vi "Init CAN Drive.vi"(0 "Front Left Motor Device Number":u8=1, 1 "refnum name":string="robotDrive", 2 "Encoder Codes Per Rev":u16=250, 5 "Rear Left Motor Device Number":u8=2, 7 "Front Right Motor Device Number":u8=3, 9 "Rear Right Motor Device Number":u8=4, 11 "error in (no error)":errorcluster, 12 "Invert":bool=TRUE) -> (15 "error out":errorcluster)   [LabVIEW 2012]
uses:
  <vilib>/Rock Robotics/WPI/CAN/Jaguar/SubVIs/WPI_CANJaguar_ControlMode.ctl
  <vilib>/Rock Robotics/WPI/CAN/Jaguar/SubVIs/WPI_CANJaguar_BrakeCoastMode.ctl
  <vilib>/Rock Robotics/WPI/CAN/Jaguar/SubVIs/WPI_CANJaguar_SpeedReference.ctl
  <vilib>/Rock Robotics/WPI/SafetyOutput/WPI_SafetyOutputConfigMenu.ctl
  <vilib>/Rock Robotics/WPI/MotorControl/WPI_MotorControlOpenCANJaguar.vi
  <vilib>/Rock Robotics/WPI/RobotDrive/WPI_RobotDriveOpen4MotorWithExistingMotors.vi
panel:
  in  "Control Mode":T1
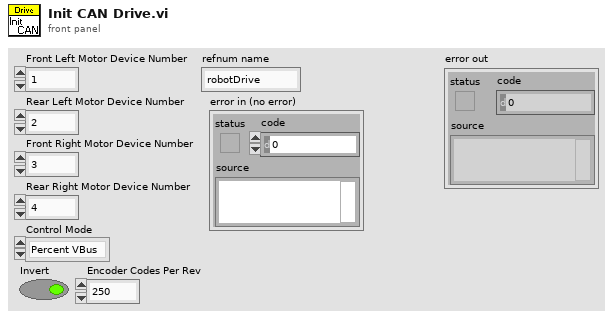
[diagram p1: front panel]
types:
  T1 = typedef "WPI_CANJaguar_ControlMode.ctl" = enum8{"Percent VBus", "Current", "Speed", "Position", "Voltage"}
  T2 = typedef "WPI_SafetyOutputConfigMenu.ctl" = enum16{"Enable", "Disable"}
  T3 = typedef "WPI_CANJaguar_SpeedReference.ctl" = u8
  T4 = typedef "WPI_CANJaguar_BrakeCoastMode.ctl" = enum8{"Jumper", "Brake", "Coast"}
  T5 = typedef "WPI_MotorControlDeviceRef.ctl" = cluster{"DeviceStatus":errorcluster, "Type":enum16{"PWM", "CAN"}, "PWM":cluster{"Digital Module":T6, "PWM Channel":T7, "DeadBand":T8}, "CAN":cluster{"Device Number":u8, "Control Mode":T1, "Semaphore":T9, "Max Vout":dbl}, "Invert":bool, "TransformRef":T10, "InvTransformRef":T10}
  T6 = typedef "FPGA_TypedefDigitalModule.ctl" = enum16{"Digital Module 1", "Digital Module 2"}
  T7 = typedef "FPGA_DIOPWMChannel.ctl" = enum8{"PWM 1", "PWM 2", "PWM 3", "PWM 4", "PWM 5", "PWM 6", "PWM 7", "PWM 8", "PWM 9", "PWM 10", "Invalid"}
  T8 = typedef "WPI_PWMDeadband.ctl" = cluster{"Name":string, "maxPositivePwm":i32, "minPositivePwm":i32, "centerPwm":i32, "maxNegativePwm":i32, "minNegativePwm":i32, "angularRange":u16}
  T9 = typedef "Semaphore RefNum" = refnum<k1>
  T10 = typedef "WPI_PWMTransform_ConPane.ctl" = refnum<vi>
  T11 = typedef "WPI_RobotDriveDevRef.ctl" = cluster{"DevStatus":errorcluster, "Motors[]":T5[], "Square Inputs":bool, "Max Output":dbl, "Isochronous":bool}
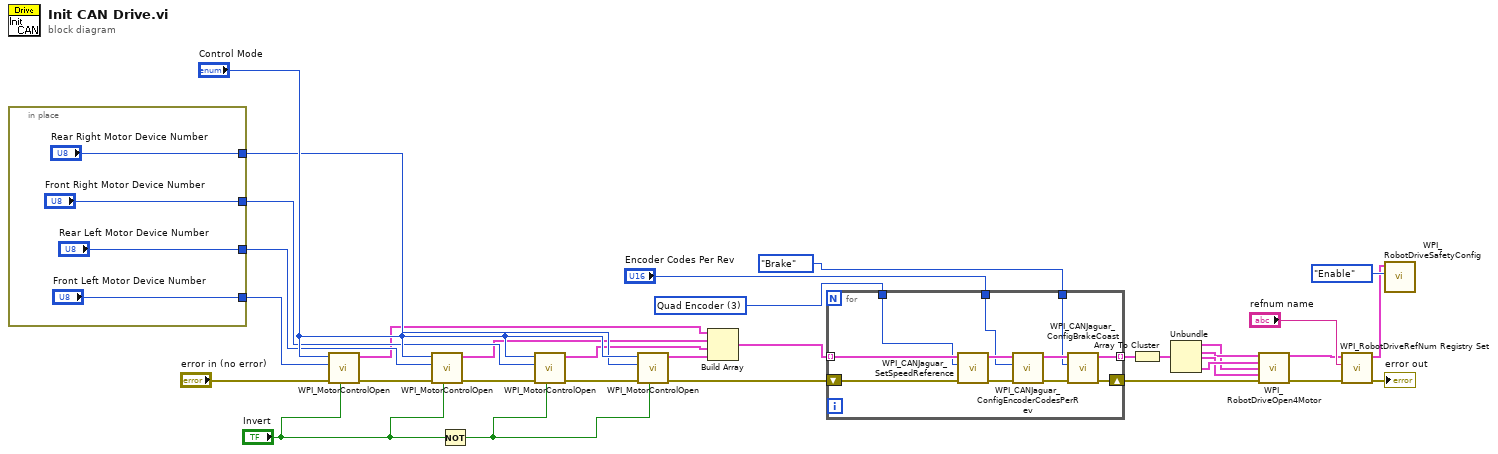
[diagram p0: block diagram]
diagram:
  w5 = T3 3 items=["Encoder"=0, "Inv Encoder"=2, "Quad Encoder"=3, "None"=255] ("Speed Reference")
  n1 = in-place {
    in-place-border: ["Front Left Motor Device Number"] -> w32
    in-place-border: ["Rear Left Motor Device Number"] -> w31
    in-place-border: ["Rear Right Motor Device Number"] -> w30
    in-place-border: ["Front Right Motor Device Number"] -> w29
  }
  n2 = call-poly <vilib>:"WPI_MotorControlOpen.vi"("Invert"="Invert", "error in (no error)"="error in (no error)", "Device Number"=w32, "Control Mode"="Control Mode") -> ("error out"=w26:errorcluster, "MotorControlDeviceRef"=w23:T5)  [unwired: 6 in]
  n3 = call-poly <vilib>:"WPI_MotorControlOpen.vi"("Invert"="Invert", "error in (no error)"=w26, "Device Number"=w31, "Control Mode"="Control Mode") -> ("error out"=w25:errorcluster, "MotorControlDeviceRef"=w22:T5)  [unwired: 6 in]
  n4 = Not(x="Invert") -> (.not. x?=w27:bool)
  n5 = call-poly <vilib>:"WPI_MotorControlOpen.vi"("Invert"=w27, "error in (no error)"=w25, "Device Number"=w29, "Control Mode"="Control Mode") -> ("error out"=w24:errorcluster, "MotorControlDeviceRef"=w21:T5)  [unwired: 6 in]
  n6 = call-poly <vilib>:"WPI_MotorControlOpen.vi"("Invert"=w27, "error in (no error)"=w24, "Device Number"=w30, "Control Mode"="Control Mode") -> ("error out"=w9:errorcluster, "MotorControlDeviceRef"=w20:T5)  [unwired: 6 in]
  n7 = Build Array(w23, w22, w21, w20) -> (w18:T5[])
  n8 = for {
    tunnel: w18 -> [w46] mode=indexing
    tunnel: [w48] -> w17 mode=indexing
    shift-right: [w47] -> w8
    shift-left: w9 -> [w45]
    tunnel: "Encoder Codes Per Rev" -> [w40]
    tunnel: WPI_CANJaguar_BrakeCoastMode."Brake" ("Brake / Coast Mode") -> [w39]
    tunnel: w5 -> [w38]
    n9 = call <vilib>:"WPI_CANJaguar_SetSpeedReference.vi"("error in (no error)"=w45, "Speed Reference"=w38, "CAN Jaguar Ref"=w46) -> ("error out"=w44:errorcluster, "CAN Jaguar Ref Out"=w43:T5)  [unwired: 7 in]
    n10 = call <vilib>:"WPI_CANJaguar_ConfigEncoderCodesPerRev.vi"("error in (no error)"=w44, "Encoder Codes Per Rev"=w40, "CAN Jaguar Ref"=w43) -> ("error out"=w41:errorcluster, "CAN Jaguar Ref Out"=w42:T5)  [unwired: 7 in]
    n11 = call <vilib>:"WPI_CANJaguar_ConfigBrakeCoast.vi"("error in (no error)"=w41, "Brake / Coast Mode"=w39, "CAN Jaguar Ref"=w42) -> ("error out"=w47:errorcluster, "CAN Jaguar Ref Out"=w48:T5)  [unwired: 7 in]
  }
  n12 = Array To Cluster(array=w17) -> (cluster=w16:cluster{"[0]":T5, "[1]":T5, "[2]":T5, "[3]":T5})
  n13 = Unbundle(w16) -> ("[0]"=w10:T5, "[1]"=w11:T5, "[2]"=w12:T5, "[3]"=w13:T5)
  n14 = call-poly <vilib>:"WPI_RobotDriveOpen4Motor.vi"("Rear Left Motor Dev Ref"=w11, "Rear Right Motor Dev Ref"=w13, "Front Left Motor Dev Ref"=w10, "Front Right Motor Dev Ref"=w12, "error in (no error)"=w8) -> ("RobotDriveDevRef"=w14:T11, "error out"=w15:errorcluster)  [unwired: 9 in]
  n15 = call <vilib>:"WPI_RobotDriveRefNum Registry Set.vi"("error in (no error)"=w15, "refnum name"="refnum name", "RobotDriveDevRef"=w14) -> ("error out"=→"error out":errorcluster, "RobotDriveDevRef"=w1:T11)  [unwired: 7 in]
  n16 = call <vilib>:"WPI_RobotDriveSafetyConfig.vi"("mode"=WPI_SafetyOutputConfigMenu."Enable", "RobotDriveDevRef"=w1) -> ()  [unwired: 8 in, 2 out]
